vi "Show Actions Updated Dialog If Necessary.vi"(11 "Steps with updated actions":string[](array[string])) -> ()   [LabVIEW 2020, in "Output Sequencer.lvlib" / "Settings UI.lvclass"]
uses:
  Settings UI.lvclass
  Globals/Dialog Strings.vi
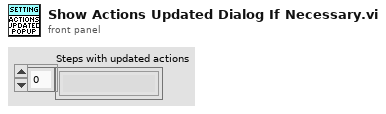
[diagram p1: front panel]
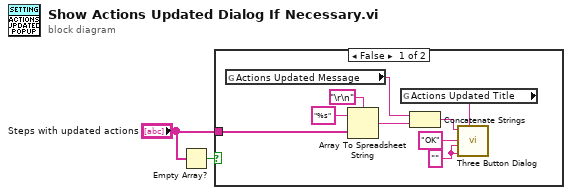
[diagram p0: block diagram]
diagram:
  n1 = Empty Array?(array="Steps with updated actions") -> (empty?=w1:bool)
  n2 = case shown="False" w1 {
    tunnel: "Steps with updated actions" -> [w8 _]
    frame False {
      w11 = "" ("Right Button Text (\"Cancel\")")
      n3 = global read "Dialog Strings.vi" "Actions Updated Message"() -> (w5:string)
      n4 = Array To Spreadsheet String(delimiter (Tab)="\r\n", array=w8, 3:"%s" ("format string")) -> (spreadsheet string=w7:string)
      n5 = global read "Dialog Strings.vi" "Actions Updated Title"() -> (w4:string)
      n6 = Concatenate Strings(w5, w7) -> (w6:string)
      n7 = call <vilib>:"Three Button Dialog.vi"("Window Title (\"\")"=w4, "Right Button Text (\"Cancel\")"=w11, "Center Button Text (\"No\")"=w11, "Left Button Text (\"Yes\")"="OK" ("Left Button Text (\"Yes\")"), "message"=w6) -> ()  [unwired: 6 in, 1 out]
    }
    frame True {
    }
  }
